vi "Untitled 1.vi"(7 "OPERACIONES":T2(ring), 8 "Error In":errorcluster, 10 "OPERADORES":T1 {"y 2" scale=0.0..4.0; "Meter" scale=-360.0..360.0 scale format="%#_3g"; "y" scale=-150.0..150.0; "x" scale=-150.0..150.0}, 11 "IMAGEN 1":path) -> (0 "Error Out":errorcluster, 1 "HISTOGRAMA":dbl[][](graph), 2 "IMAGEN MODIFICADA":picture, 3 "IMAGEN ORIGINAL":picture)   [LabVIEW 2016]
uses:
  <vilib>/picture/picture.llb/Draw True-Color Pixmap.vi
  <vilib>/imath/engines/lvmath2/RunTimeEngine/Managers/WorkSpace/UID Generator.vi
  <vilib>/imath/engines/lvmath2/RunTimeEngine/BuiltInFunctions/size/NIMS_[I32,I32]=size(GM).vi
  <instcachedir>/0/NIMS_[I32,I32]=size(GM)_B0A6EC1255BB4C8AB801FE6F734128D9.lvgen/NIMS_[I32,I32]=size(GM)_B0A6EC1255BB4C8AB801FE6F734128D9_005.vi
  <vilib>/imath/engines/lvmath2/RunTimeSupport/NIMS_Complex To Real.vi
  <instcachedir>/0/NIMS_Complex To Real_A9DD49CC305F495FA24B9F5762C73A31.lvgen/NIMS_Complex To Real_A9DD49CC305F495FA24B9F5762C73A31_001.vi
  <vilib>/imath/engines/lvmath2/RunTimeEngine/BuiltInFunctions/zeros/NIMS_M=zeros(I32,I32).vi
  <vilib>/imath/engines/lvmath2/RunTimeEngine/ErrorHandling/NIMS_Create Error From Enums.vi
  <vilib>/imath/engines/lvmath2/RunTimeEngine/RangeToken/NIMS_Range.vi
  <instcachedir>/0/NIMS_Range_A7C094595B484CA7AF10685B02D808ED.lvgen/NIMS_Range_A7C094595B484CA7AF10685B02D808ED_000.vi
  <vilib>/imath/engines/lvmath2/RunTimeSupport/NIMS_Error if Not Equal.vi
  <instcachedir>/0/NIMS_Error if Not Equal_43252A79AD05436189442EC0C5E5AB8A.lvgen/NIMS_Error if Not Equal_43252A79AD05436189442EC0C5E5AB8A_001.vi
  <vilib>/imath/engines/lvmath2/RunTimeEngine/IndexReplace/NIMS M(V,V)=M.vi
  <instcachedir>/0/NIMS M(V,V)=M_7C673E496ABD4677A4D7F51E7F4F45D1.lvgen/NIMS M(V,V)=M_7C673E496ABD4677A4D7F51E7F4F45D1_004.vi
  <vilib>/imath/engines/lvmath2/RunTimeEngine/BuiltInFunctions/size/NIMS_I32=size(GM,I32).vi
  <instcachedir>/0/NIMS_I32=size(GM,I32)_122058B1B3294FAEA5DC209B92B394E4.lvgen/NIMS_I32=size(GM,I32)_122058B1B3294FAEA5DC209B92B394E4_005.vi
  <vilib>/imathl/engines/lvmath/Functions/Error Handling/Create Error.vi
  <vilib>/imath/engines/lvmath2/RunTimeEngine/BuiltInFunctions/size/NIMS_I32Row=size(GM).vi
  <instcachedir>/0/NIMS_I32Row=size(GM)_10ACDCB9F1F84A7E9F42C91D87611FB5.lvgen/NIMS_I32Row=size(GM)_10ACDCB9F1F84A7E9F42C91D87611FB5_006.vi
  <vilib>/imath/engines/lvmath2/RunTimeEngine/BuiltInFunctions/zeros/NIMS_M=zeros(I32V).vi
  <vilib>/imath/engines/lvmath2/RunTimeEngine/RangeToken/NIMS_Range_R2 - Integer.vi
  <instcachedir>/0/NIMS_Range_R2 - Integer_89B873E74E6E489885E44F751DD9C6BF.lvgen/NIMS_Range_R2 - Integer_89B873E74E6E489885E44F751DD9C6BF_000.vi
  <vilib>/imath/engines/lvmath2/RunTimeEngine/CommandStatement/MC_CommandStatement_break.vi
  <vilib>/imath/engines/lvmath2/RunTimeEngine/BuiltInFunctions/round/NIMS_round(DBL-S).vi
  <instcachedir>/0/NIMS_Error if Not Equal_43252A79AD05436189442EC0C5E5AB8A.lvgen/NIMS_Error if Not Equal_43252A79AD05436189442EC0C5E5AB8A_000.vi
  <vilib>/imath/engines/lvmath2/RunTimeEngine/IndexRead/NIMS M(S,S).vi
  <instcachedir>/0/NIMS M(S,S)_AC51E74150A542F7991B9634C66F3096.lvgen/NIMS M(S,S)_AC51E74150A542F7991B9634C66F3096_002.vi
  <vilib>/imath/engines/lvmath2/RunTimeEngine/IndexReplace/NIMS M(S,S)=S.vi
  <instcachedir>/0/NIMS M(S,S)=S_98E40400474E4398B113AE20298B4F82.lvgen/NIMS M(S,S)=S_98E40400474E4398B113AE20298B4F82_003.vi
  <vilib>/imath/engines/lvmath2/RunTimeEngine/RunTimeType/NIMS_RunTimeType_From StrictType (excl LVString).vi
  <instcachedir>/0/NIMS_RunTimeType_From StrictType (excl LVString)_BBF44FB49F834B71AF7A14CCEDF8BECD.lvgen/NIMS_RunTimeType_From StrictType (excl LVString)_BBF44FB49F834B71AF7A14CCEDF8BECD_000.vi
  <vilib>/imath/engines/lvmath2/RunTimeEngine/LocalVariableDefStatement/MC_LocalVariableDefStatement_Display.vi
  <vilib>/imath/engines/lvmath2/RunTimeEngine/Managers/SymbolTable/Clear UID.vi
  <vilib>/imath/engines/lvmath2/RunTimeEngine/NodeEndStatement/NIMS_NodeEndStatement_Output.vi
  <instcachedir>/0/NIMS_NodeEndStatement_Output_53EC0D466D134D7ABD903AC30B43404B.lvgen/NIMS_NodeEndStatement_Output_53EC0D466D134D7ABD903AC30B43404B_001.vi
  <instcachedir>/0/NIMS_NodeEndStatement_Output_53EC0D466D134D7ABD903AC30B43404B.lvgen/NIMS_NodeEndStatement_Output_53EC0D466D134D7ABD903AC30B43404B_010.vi
  <vilib>/imath/engines/lvmath2/RunTimeEngine/ErrorHandling/NIMS_Finalize Error.vi
  <vilib>/Analysis/Matrix/Numeric/Conversions/Array To Matrix - RA2.vi
  <vilib>/Analysis/Matrix/Numeric/Conversions/Matrix To Array - RM.vi
  <vilib>/imath/engines/lvmath2/RunTimeEngine/BuiltInFunctions/rotate90/NIMS_rotate90.vi
  <instcachedir>/0/NIMS_rotate90_7DC1660D109944E092D2EB6E3185A1B6.lvgen/NIMS_rotate90_7DC1660D109944E092D2EB6E3185A1B6_004.vi
  <vilib>/imath/engines/lvmath2/RunTimeEngine/IndexRead/NIMS M(R2,S).vi
  <instcachedir>/0/NIMS M(R2,S)_56813DCFDD5A484292D2195AF15D2BF5.lvgen/NIMS M(R2,S)_56813DCFDD5A484292D2195AF15D2BF5_000.vi
  <vilib>/imath/engines/lvmath2/RunTimeEngine/IndexReplace/NIMS M(R2,S)=V.vi
  <instcachedir>/0/NIMS M(R2,S)=V_4CAA475A15784754AE70E3CCB958AE2E.lvgen/NIMS M(R2,S)=V_4CAA475A15784754AE70E3CCB958AE2E_000.vi
  <instcachedir>/0/NIMS_NodeEndStatement_Output_53EC0D466D134D7ABD903AC30B43404B.lvgen/NIMS_NodeEndStatement_Output_53EC0D466D134D7ABD903AC30B43404B_002.vi
  <instcachedir>/0/NIMS M(S,S)_AC51E74150A542F7991B9634C66F3096.lvgen/NIMS M(S,S)_AC51E74150A542F7991B9634C66F3096_003.vi
  <instcachedir>/0/NIMS M(S,S)_AC51E74150A542F7991B9634C66F3096.lvgen/NIMS M(S,S)_AC51E74150A542F7991B9634C66F3096_000.vi
  <instcachedir>/0/NIMS M(S,S)=S_98E40400474E4398B113AE20298B4F82.lvgen/NIMS M(S,S)=S_98E40400474E4398B113AE20298B4F82_000.vi
  <vilib>/Analysis/Matrix/NI_Matrix.lvlib
  <vilib>/imath/engines/lvmath2/RunTimeEngine/Managers/SymbolTable/NIMS_WorkSpace.lvlib
panel:
  out "size(s)":i32[](array[numeric])
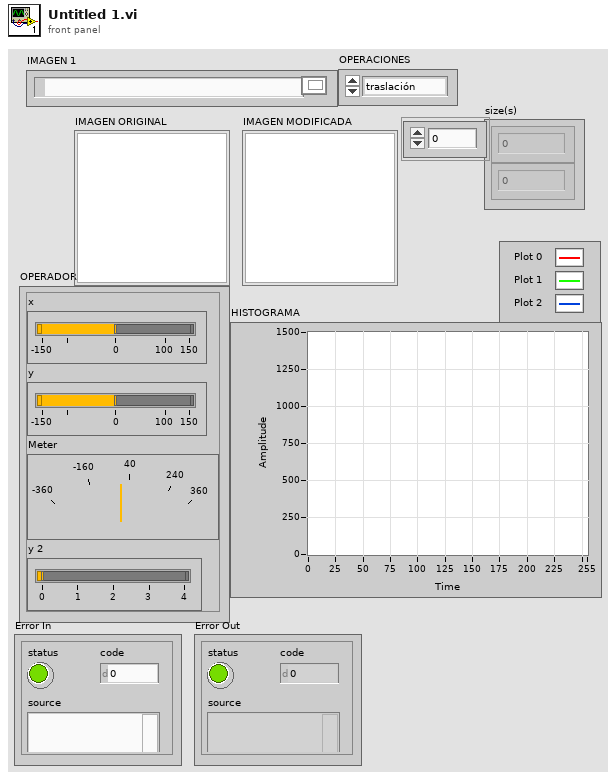
[diagram p1: front panel]
types:
  T1 = cluster{"x":dbl, "y":dbl, "Meter":dbl, "y 2":i64}
  T2 = enum16{"traslación", "Rotación", "Zoom", "GIROH", "GIROV", "Extracción", "Sustitución", "UNION"}
  T3 = typedef "imagedata.ctl" = cluster{"image type":i32, "image depth":i32, "image":u8[], "mask":u8[], "colors":u32[], "Rectangle":cluster{"left":i16, "top":i16, "right":i16, "bottom":i16}}
  T4 = typedef "NI_Matrix.lvlib/RealMatrix.ctl" = dbl[][]
  T5 = cluster{"left":i16, "top":i16, "right":i16, "bottom":i16}
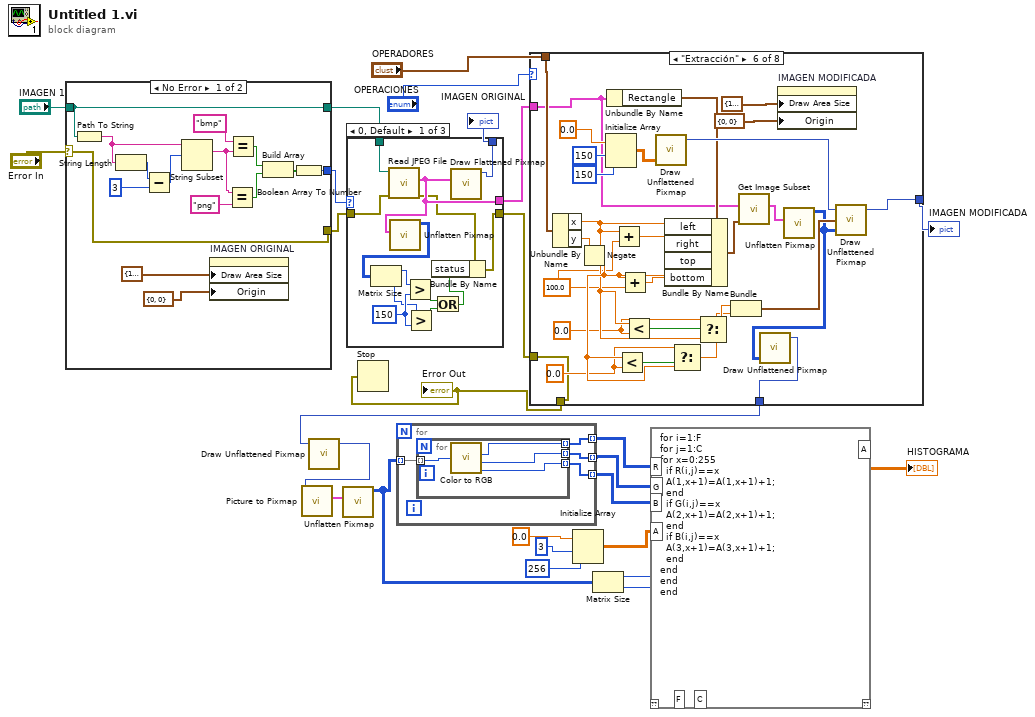
[diagram p0: block diagram]
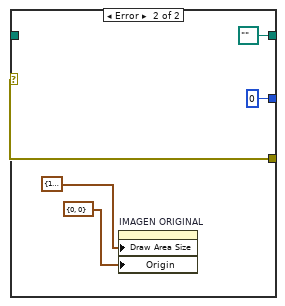
[diagram p2: hidden frame]
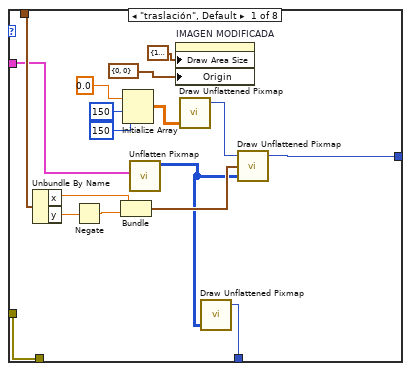
[diagram p3: hidden frame]
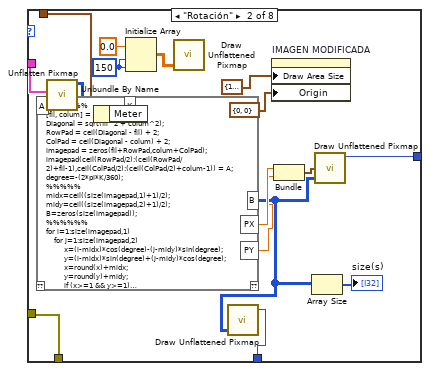
[diagram p4: hidden frame]
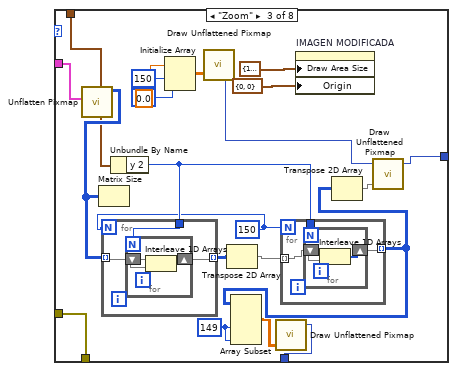
[diagram p5: hidden frame]
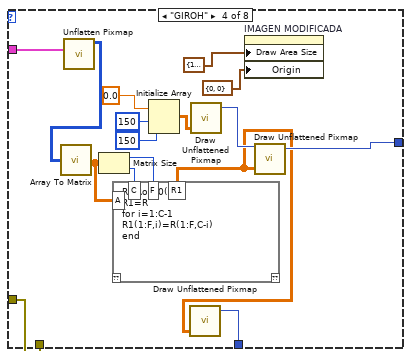
[diagram p6: hidden frame]
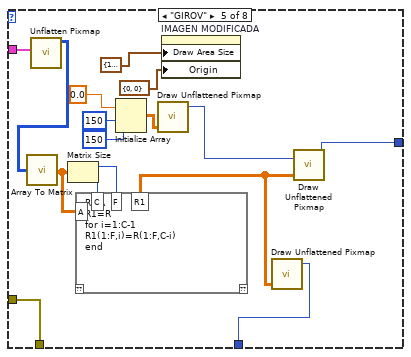
[diagram p7: hidden frame]
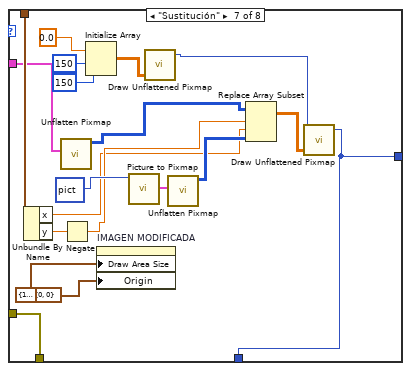
[diagram p8: hidden frame]
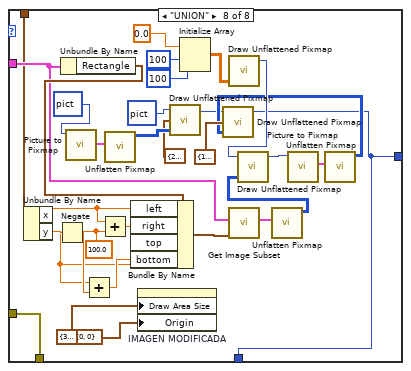
[diagram p9: hidden frame]
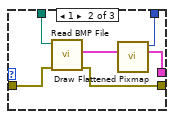
[diagram p10: hidden frame]
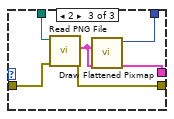
[diagram p11: hidden frame]
diagram:
  n1 = case shown="No Error" "Error In" {
    selector: "Error In" -> [w30 w46]
    tunnel: [w36 u32 0] -> w26
    tunnel: [w29 path "" ("File Path Control")] -> w25
    tunnel: [w30 w46] -> w24
    tunnel: "IMAGEN 1" -> [w29 _]
    frame No Error {
      n2 = Path To String(path=w29) -> (string=w31:string)
      n3 = String Length(string=w31) -> (length=w41:i32)
      n4 = Subtract(x=w41, y=3) -> (x-y=w39:i32)
      n5 = String Subset(string=w31, offset (0)=w39) -> (substring=w32:string)  [unwired: 1 in]
      n6 = property on="IMAGEN ORIGINAL" class="Pict"("Draw Area Size"=cluster{"Width":u32, "Height":u32} {"Width"=150, "Height"=150} ("Caption.Size"), "Origin"=cluster{"Horizontal":i16, "Vertical":i16} {"Horizontal"=0, "Vertical"=0}) -> ()  [unwired: 2 in, 2 out]
      n7 = Equal?(x=w32, y="png" ("x")) -> (x = y?=w34:bool)
      n8 = Equal?(x="bmp", y=w32) -> (x = y?=w33:bool)
      n9 = Build Array(w33, w34) -> (w35:bool[])
      n10 = Boolean Array To Number(Boolean array=w35) -> (number=w36:u32)
    }
    frame Error {
      n11 = property on="IMAGEN ORIGINAL" class="Pict"("Draw Area Size"=cluster{"Width":u32, "Height":u32} {"Width"=150, "Height"=150} ("Caption.Size"), "Origin"=cluster{"Horizontal":i16, "Vertical":i16} {"Horizontal"=0, "Vertical"=0}) -> ()  [unwired: 2 in, 2 out]
    }
  }
  n12 = case shown="0, Default" w26 {
    tunnel: w25 -> [w59 w64 w69]
    tunnel: [w56 w63 w68] -> w21
    tunnel: w24 -> [w58 w62 w67]
    tunnel: [w47 w61 w66] -> w16
    tunnel: [w57 w60 w65] -> w20
    frame 0, Default {
      w52 = 150 ("y")
      n13 = call <vilib>:"Read JPEG File.vi"("error in (no error)"=w58, "path to JPEG file"=w59) -> ("error out"=w48:errorcluster, "image data"=w56:T3)  [unwired: 7 in, 1 out]
      n14 = call <vilib>:"Unflatten Pixmap.vi"("image data"=w56) -> ("24-bit pixmap"=w55:u32[][])  [unwired: 4 in, 6 out]
      n15 = Matrix Size(0:w55) -> (1:w51:i32, 2:w50:i32)
      n16 = Greater?(x=w51, y=w52) -> (0:w53:bool)
      n17 = Greater?(x=w50, y=w52) -> (0:w54:bool)
      n18 = Or(x=w53, y=w54) -> (x .or. y?=w49:bool)
      n19 = Bundle By Name(cluster=w48, "status"=w49) -> (w47:errorcluster)
      n20 = call <vilib>:"Draw Flattened Pixmap.vi"("image data"=w56) -> ("new picture"=w57:picture)  [unwired: 8 in]
    }
    frame 1 {
      n21 = call <vilib>:"Read BMP File.vi"("error in (no error)"=w62, "path to BMP file"=w64) -> ("error out"=w61:errorcluster, "image data"=w63:T3)  [unwired: 7 in, 1 out]
      n22 = call <vilib>:"Draw Flattened Pixmap.vi"("image data"=w63) -> ("new picture"=w60:picture)  [unwired: 8 in]
    }
    frame 2 {
      n23 = call <vilib>:"Read PNG File.vi"("error in (no error)"=w67, "path to PNG file"=w69) -> ("error out"=w66:errorcluster, "image data"=w68:T3)  [unwired: 7 in, 1 out]
      n24 = call <vilib>:"Draw Flattened Pixmap.vi"("image data"=w68) -> ("new picture"=w65:picture)  [unwired: 8 in]
    }
  }
  "IMAGEN ORIGINAL" <- w20
  n25 = case shown="\"Extracción\"" "OPERACIONES" {
    tunnel: [w83 w103 w633 w663 w828 w966 w995 w1012] -> w19
    tunnel: w21 -> [w78 w101 w634 w662 w822 w967 w1002 w1040]
    tunnel: "OPERADORES" -> [w80 w102 w635 _ _ w968 w1011 w1036]
    tunnel: w16 -> [w77 w98 w647 w673 w815 w969 w1001 w1013]
    tunnel: [w77 w98 w647 w673 w815 w969 w1001 w1013] -> w15
    tunnel: [w70 w92 w632 w660 w813 w964 w995 w1012] -> w14
    frame "traslación", Default {
      n26 = Unbundle By Name(w80) -> ("x"=w79:dbl, "y"=w74:dbl)
      n27 = Negate(x=w74) -> (-x=w73:dbl)
      n28 = Bundle("x"=w79, w73) -> (w72:cluster{"x":dbl, dbl})  [unwired: 1 in]
      n29 = Initialize Array(0.0 ("element"), 150 ("dimension size"), 150 ("dimension size")) -> (w82:dbl[][])
      n30 = call <vilib>:"Unflatten Pixmap.vi"("image data"=w78) -> ("24-bit pixmap"=w71:u32[][])  [unwired: 4 in, 6 out]
      n31 = property on="IMAGEN MODIFICADA" class="Pict"("Draw Area Size"=cluster{"Width":u32, "Height":u32} {"Width"=150, "Height"=150} ("Caption.Size"), "Origin"=cluster{"Horizontal":i16, "Vertical":i16} {"Horizontal"=0, "Vertical"=0}) -> ()  [unwired: 2 in, 2 out]
      n32 = call-poly <vilib>:"Draw Unflattened Pixmap.vi"("data (RGB format)"=w82) -> ("new picture"=w81:picture)  [unwired: 8 in]
      n33 = call-poly <vilib>:"Draw Unflattened Pixmap.vi"("data (RGB format)"=w71) -> ("new picture"=w70:picture)  [unwired: 8 in]
      n34 = call-poly <vilib>:"Draw Unflattened Pixmap.vi"("picture"=w81, "top left point(0, 0)"=w72, "data (RGB format)"=w71) -> ("new picture"=w83:picture)  [unwired: 6 in]
    }
    frame "Rotación" {
      w97 = 150 ("dimension size")
      n35 = call <vilib>:"Unflatten Pixmap.vi"("image data"=w101) -> ("24-bit pixmap"=w93:u32[][])  [unwired: 4 in, 6 out]
      n36 = Unbundle By Name(w102) -> ("Meter"=w94:dbl)
      n37 = mathscript code="%%%%%%\n[fil, colum] = size(A); \nDiagonal = sqrt(fil^2 + colum^2); \nRowPad = ceil(Diagonal - fil) + 2;\nColPad = ceil(Diagonal - colum) + 2;\nimagepad = zeros(fil+RowPad,colum+ColPad);\nimagepad(ceil(RowPad/2):(ceil(RowPad/2)+fil-1),ceil(ColPad/2):(ceil(ColPad/2)+colum-1)) = A;\ndegree=-(2*pi*K/360);\n%%%%%\nmidx=ceil((size(imagepad,1)+1)/2);\nmidy=ceil((size(imagepad,2)+1)/2);\nB=zeros(size(imagepad));\n%%%%%%\nfor i=1:size(imagepad,1)\n    for j=1:size(imagepad,2)\n         x=(i-midx)*cos(degree)-(j-midy)*sin(degree);\n         y=(i-midx)*sin(degree)+(j-midy)*cos(degree);\n         x=round(x)+midx;\n         y=round(y)+midy;\n         if (x>=1 && y>=1)\n             B(x,y)=imagepad(i,j);        \n         end\n    end\nend\n[m,n]=size(B)\nPY=-(midy/2)-2\nPX=-(midx/8)-2"("K"=w94, "A"=w93) -> ("B"=w88:u32[][], "PX"=w90:dbl, "PY"=w89:dbl)  [unwired: 1 in, 1 out]
      n38 = Initialize Array(0.0 ("element"), w97, w97) -> (w95:dbl[][])
      n39 = call-poly <vilib>:"Draw Unflattened Pixmap.vi"("data (RGB format)"=w95) -> ()  [unwired: 8 in, 1 out]
      n40 = call-poly <vilib>:"Draw Unflattened Pixmap.vi"("data (RGB format)"=w88) -> ("new picture"=w92:picture)  [unwired: 8 in]
      n41 = property on="IMAGEN MODIFICADA" class="Pict"("Draw Area Size"=cluster{"Width":u32, "Height":u32} {"Width"=150, "Height"=150} ("Caption.Size"), "Origin"=cluster{"Horizontal":i16, "Vertical":i16} {"Horizontal"=0, "Vertical"=0}) -> ()  [unwired: 2 in, 2 out]
      n42 = Bundle("PX"=w90, "PY"=w89) -> (w91:cluster{"PX":dbl, "PY":dbl})  [unwired: 1 in]
      n43 = Array Size(array=w88) -> (size(s)=→"size(s)":i32[])
      n44 = call-poly <vilib>:"Draw Unflattened Pixmap.vi"("top left point(0, 0)"=w91, "data (RGB format)"=w88) -> ("new picture"=w103:picture)  [unwired: 7 in]
    }
    frame "Zoom" {
      w629 = 149 ("row N")
      w637 = 150
      n45 = call <vilib>:"Unflatten Pixmap.vi"("image data"=w634) -> ("24-bit pixmap"=w636:u32[][])  [unwired: 4 in, 6 out]
      n46 = Matrix Size(0:w636) -> ()  [unwired: 2 out]
      n47 = Unbundle By Name(w635) -> ("y 2"=w639:i64)
      n48 = for {
        N: w637 -> [_]
        tunnel: w636 -> [w657] mode=indexing
        tunnel: w639 -> [w656]
        tunnel: [w655] -> w641 mode=indexing
        n49 = for {
          N: w656 -> [_]
          shift-right: [w658] -> w655
          shift-left: w657 -> [w659]
          n50 = Interleave 1D Arrays(w659, w659) -> (w658:u32[])
        }
      }
      n51 = Initialize Array(0.0 ("element"), 150 ("dimension size"), 150 ("dimension size")) -> (w643:dbl[][])
      n52 = call-poly <vilib>:"Draw Unflattened Pixmap.vi"("data (RGB format)"=w643) -> ("new picture"=w642:picture)  [unwired: 8 in]
      n53 = Transpose 2D Array(2D array=w641) -> (transposed array=w640:u32[][])
      n54 = for {
        N: w637 -> [_]
        tunnel: w639 -> [w652]
        tunnel: [w651] -> w631 mode=indexing
        tunnel: w640 -> [w650] mode=indexing
        n55 = for {
          N: w652 -> [_]
          shift-right: [w653] -> w651
          shift-left: w650 -> [w654]
          n56 = Interleave 1D Arrays(w654, w654) -> (w653:u32[])
        }
      }
      n57 = Array Subset(array=w631, length (row)=w629, length (col)=w629) -> (w630:dbl[][])  [unwired: 2 in]
      n58 = call-poly <vilib>:"Draw Unflattened Pixmap.vi"("data (RGB format)"=w630) -> ("new picture"=w632:picture)  [unwired: 8 in]
      n59 = property on="IMAGEN MODIFICADA" class="Pict"("Draw Area Size"=cluster{"Width":u32, "Height":u32} {"Width"=150, "Height"=150} ("Caption.Size"), "Origin"=cluster{"Horizontal":i16, "Vertical":i16} {"Horizontal"=0, "Vertical"=0}) -> ()  [unwired: 2 in, 2 out]
      n60 = Transpose 2D Array(2D array=w631) -> (transposed array=w638:u32[][])
      n61 = call-poly <vilib>:"Draw Unflattened Pixmap.vi"("picture"=w642, "data (RGB format)"=w638) -> ("new picture"=w633:picture)  [unwired: 7 in]
    }
    frame "GIROH" {
      n62 = call <vilib>:"Unflatten Pixmap.vi"("image data"=w662) -> ("24-bit pixmap"=w667:u32[][])  [unwired: 4 in, 6 out]
      n63 = call-poly <vilib>:"Array To Matrix.vi"("Real 2D Array"=w667) -> ("Real Matrix"=w664:T4)
      n64 = Matrix Size(0:w664) -> (1:w665:i32, 2:w672:i32)
      n65 = mathscript code="R=Rot90(A,2)\nR1=R\nfor i=1:C-1\nR1(1:F,i)=R(1:F,C-i)\nend"("A"=w664, "C"=w672, "F"=w665) -> ("R1"=w661:dbl[][])  [unwired: 1 in, 1 out]
      n66 = Initialize Array(0.0 ("element"), 150 ("dimension size"), 150 ("dimension size")) -> (w668:dbl[][])
      n67 = call-poly <vilib>:"Draw Unflattened Pixmap.vi"("data (RGB format)"=w661) -> ("new picture"=w660:picture)  [unwired: 8 in]
      n68 = call-poly <vilib>:"Draw Unflattened Pixmap.vi"("data (RGB format)"=w668) -> ("new picture"=w666:picture)  [unwired: 8 in]
      n69 = property on="IMAGEN MODIFICADA" class="Pict"("Draw Area Size"=cluster{"Width":u32, "Height":u32} {"Width"=150, "Height"=150} ("Caption.Size"), "Origin"=cluster{"Horizontal":i16, "Vertical":i16} {"Horizontal"=0, "Vertical"=0}) -> ()  [unwired: 2 in, 2 out]
      n70 = call-poly <vilib>:"Draw Unflattened Pixmap.vi"("picture"=w666, "data (RGB format)"=w661) -> ("new picture"=w663:picture)  [unwired: 7 in]
    }
    frame "GIROV" {
      n71 = call <vilib>:"Unflatten Pixmap.vi"("image data"=w822) -> ("24-bit pixmap"=w821:u32[][])  [unwired: 4 in, 6 out]
      n72 = call-poly <vilib>:"Array To Matrix.vi"("Real 2D Array"=w821) -> ("Real Matrix"=w818:T4)
      n73 = Matrix Size(0:w818) -> (1:w819:i32, 2:w827:i32)
      n74 = mathscript code="R=A\nR1=R\nfor i=1:C-1\nR1(1:F,i)=R(1:F,C-i)\nend"("A"=w818, "C"=w827, "F"=w819) -> ("R1"=w814:dbl[][])  [unwired: 1 in, 1 out]
      n75 = Initialize Array(0.0 ("element"), 150 ("dimension size"), 150 ("dimension size")) -> (w823:dbl[][])
      n76 = call-poly <vilib>:"Draw Unflattened Pixmap.vi"("data (RGB format)"=w823) -> ("new picture"=w820:picture)  [unwired: 8 in]
      n77 = property on="IMAGEN MODIFICADA" class="Pict"("Draw Area Size"=cluster{"Width":u32, "Height":u32} {"Width"=150, "Height"=150} ("Caption.Size"), "Origin"=cluster{"Horizontal":i16, "Vertical":i16} {"Horizontal"=0, "Vertical"=0}) -> ()  [unwired: 2 in, 2 out]
      n78 = call-poly <vilib>:"Draw Unflattened Pixmap.vi"("data (RGB format)"=w814) -> ("new picture"=w813:picture)  [unwired: 8 in]
      n79 = call-poly <vilib>:"Draw Unflattened Pixmap.vi"("picture"=w820, "data (RGB format)"=w814) -> ("new picture"=w828:picture)  [unwired: 7 in]
    }
    frame "Extracción" {
      w987 = 0.0 ("y")
      w986 = 0.0 ("y")
      w982 = 100.0 ("y")
      n80 = Unbundle By Name(w968) -> ("x"=w991:dbl, "y"=w984:dbl)
      n81 = Negate(x=w984) -> (-x=w992:dbl)
      n82 = Initialize Array(0.0 ("element"), 150 ("dimension size"), 150 ("dimension size")) -> (w978:dbl[][])
      n83 = Unbundle By Name(w967) -> ("Rectangle"=w970:T5)
      n84 = Add(x=w991, y=w982) -> (x+y=w973:dbl)
      n85 = Less?(x=w992, y=w986) -> (x < y?=w983:bool)
      n86 = Add(x=w992, y=w982) -> (x+y=w972:dbl)
      n87 = Less?(x=w991, y=w987) -> (x < y?=w988:bool)
      n88 = call-poly <vilib>:"Draw Unflattened Pixmap.vi"("data (RGB format)"=w978) -> ("new picture"=w979:picture)  [unwired: 8 in]
      n89 = Bundle By Name(cluster=w970, "left"=w991, "right"=w973, "top"=w992, "bottom"=w972) -> (w971:T5)
      n90 = Select(t=w986, s=w983, f=w992) -> (s? t:f=w985:dbl)
      n91 = Select(t=w987, s=w988, f=w991) -> (s? t:f=w989:dbl)
      n92 = Bundle("x"=w989, "y"=w985) -> (w990:cluster{"x":dbl, "y":dbl})  [unwired: 1 in]
      n93 = call <vilib>:"Get Image Subset.vi"("subset rect"=w971, "image data"=w967) -> ("image subset"=w974:T3)  [unwired: 4 in, 1 out]
      n94 = property on="IMAGEN MODIFICADA" class="Pict"("Draw Area Size"=cluster{"Width":u32, "Height":u32} {"Width"=150, "Height"=150} ("Caption.Size"), "Origin"=cluster{"Horizontal":i16, "Vertical":i16} {"Horizontal"=0, "Vertical"=0}) -> ()  [unwired: 2 in, 2 out]
      n95 = call <vilib>:"Unflatten Pixmap.vi"("image data"=w974) -> ("24-bit pixmap"=w965:u32[][])  [unwired: 4 in, 6 out]
      n96 = call-poly <vilib>:"Draw Unflattened Pixmap.vi"("data (RGB format)"=w965) -> ("new picture"=w964:picture)  [unwired: 8 in]
      n97 = call-poly <vilib>:"Draw Unflattened Pixmap.vi"("picture"=w979, "top left point(0, 0)"=w990, "data (RGB format)"=w965) -> ("new picture"=w966:picture)  [unwired: 6 in]
    }
    frame "Sustitución" {
      n98 = Unbundle By Name(w1011) -> ("x"=w993:dbl, "y"=w1007:dbl)
      n99 = call <vilib>:"Unflatten Pixmap.vi"("image data"=w1002) -> ("24-bit pixmap"=w999:u32[][])  [unwired: 4 in, 6 out]
      n100 = Negate(x=w1007) -> (-x=w994:dbl)
      n101 = Initialize Array(0.0 ("element"), 150 ("dimension size"), 150 ("dimension size")) -> (w1003:dbl[][])
      n102 = property on="IMAGEN MODIFICADA" class="Pict"("Draw Area Size"=cluster{"Width":u32, "Height":u32} {"Width"=150, "Height"=150} ("Caption.Size"), "Origin"=cluster{"Horizontal":i16, "Vertical":i16} {"Horizontal"=0, "Vertical"=0}) -> ()  [unwired: 2 in, 2 out]
      n103 = call <vilib>:"Picture to Pixmap.vi"("picture"=picture bytes[30030] ("IMAGEN ORIGINAL 2")) -> ("image data"=w1006:T3)  [unwired: 9 in, 1 out]
      n104 = call-poly <vilib>:"Draw Unflattened Pixmap.vi"("data (RGB format)"=w1003) -> ("new picture"=w996:picture)  [unwired: 8 in]
      n105 = call <vilib>:"Unflatten Pixmap.vi"("image data"=w1006) -> ("24-bit pixmap"=w998:u32[][])  [unwired: 4 in, 6 out]
      n106 = Replace Array Subset(array=w999, new element=w998, index (row)=w994, index (col)=w993) -> (w997:T4)
      n107 = call-poly <vilib>:"Draw Unflattened Pixmap.vi"("picture"=w996, "data (RGB format)"=w997) -> ("new picture"=w995:picture)  [unwired: 7 in]
    }
    frame "UNION" {
      w1031 = 100.0 ("y")
      n108 = Unbundle By Name(w1036) -> ("x"=w1022:dbl, "y"=w1030:dbl)
      n109 = Negate(x=w1030) -> (-x=w1023:dbl)
      n110 = Unbundle By Name(w1040) -> ("Rectangle"=w1042:T5)
      n111 = call <vilib>:"Picture to Pixmap.vi"("picture"=picture bytes[30030] ("new picture 3")) -> ("image data"=w1029:T3)  [unwired: 9 in, 1 out]
      n112 = Add(x=w1023, y=w1031) -> (x+y=w1039:dbl)
      n113 = Add(x=w1022, y=w1031) -> (x+y=w1038:dbl)
      n114 = call <vilib>:"Unflatten Pixmap.vi"("image data"=w1029) -> ("24-bit pixmap"=w1028:u32[][])  [unwired: 4 in, 6 out]
      n115 = Bundle By Name(cluster=w1042, "left"=w1022, "right"=w1038, "top"=w1023, "bottom"=w1039) -> (w1041:T5)
      n116 = property on="IMAGEN MODIFICADA" class="Pict"("Draw Area Size"=cluster{"Width":u32, "Height":u32} {"Width"=300, "Height"=100} ("Caption.Size"), "Origin"=cluster{"Horizontal":i16, "Vertical":i16} {"Horizontal"=0, "Vertical"=0}) -> ()  [unwired: 2 in, 2 out]
      n117 = call-poly <vilib>:"Draw Unflattened Pixmap.vi"("picture"=picture bytes[30030] ("new picture 3"), "top left point(0, 0)"=cluster{"x":i16, "y":i16} {"x"=200, "y"=0}, "data (RGB format)"=w1028) -> ("new picture"=w1014:picture)  [unwired: 6 in]
      n118 = Initialize Array(0.0 ("element"), 100 ("dimension size"), 100 ("dimension size")) -> (w1032:dbl[][])
      n119 = call-poly <vilib>:"Draw Unflattened Pixmap.vi"("data (RGB format)"=w1032) -> ("new picture"=w1017:picture)  [unwired: 8 in]
      n120 = call <vilib>:"Get Image Subset.vi"("subset rect"=w1041, "image data"=w1040) -> ("image subset"=w1037:T3)  [unwired: 4 in, 1 out]
      n121 = call <vilib>:"Unflatten Pixmap.vi"("image data"=w1037) -> ("24-bit pixmap"=w1018:u32[][])  [unwired: 4 in, 6 out]
      n122 = call-poly <vilib>:"Draw Unflattened Pixmap.vi"("picture"=w1017, "data (RGB format)"=w1018) -> ("new picture"=w1016:picture)  [unwired: 7 in]
      n123 = call <vilib>:"Picture to Pixmap.vi"("picture"=w1016) -> ("image data"=w1026:T3)  [unwired: 9 in, 1 out]
      n124 = call <vilib>:"Unflatten Pixmap.vi"("image data"=w1026) -> ("24-bit pixmap"=w1015:u32[][])  [unwired: 4 in, 6 out]
      n125 = call-poly <vilib>:"Draw Unflattened Pixmap.vi"("picture"=w1014, "top left point(0, 0)"=cluster{"x":i16, "y":i16} {"x"=100, "y"=0}, "data (RGB format)"=w1015) -> ("new picture"=w1012:picture)  [unwired: 6 in]
    }
  }
  "Error Out" <- w15
  "IMAGEN MODIFICADA" <- w19
  n126 = call-poly <vilib>:"Draw Unflattened Pixmap.vi"("picture"=w14) -> ("new picture"=w12:picture)  [unwired: 8 in]
  n127 = call <vilib>:"Picture to Pixmap.vi"("picture"=w12) -> ("image data"=w11:T3)  [unwired: 9 in, 1 out]
  n128 = call <vilib>:"Unflatten Pixmap.vi"("image data"=w11) -> ("24-bit pixmap"=w3:u32[][])  [unwired: 4 in, 6 out]
  n129 = Stop(stop? (T)=w15) -> ()
  n130 = for {
    tunnel: w3 -> [w1046] mode=indexing
    tunnel: [w1045] -> w9 mode=indexing
    tunnel: [w1044] -> w4 mode=indexing
    tunnel: [w1043] -> w8 mode=indexing
    n131 = for {
      tunnel: w1046 -> [w1050] mode=indexing
      tunnel: [w1049] -> w1045 mode=indexing
      tunnel: [w1048] -> w1044 mode=indexing
      tunnel: [w1047] -> w1043 mode=indexing
      n132 = call <vilib>:"Color to RGB.vi"("Color"=w1050) -> ("R"=w1049:u8, "G"=w1048:u8, "B"=w1047:u8)  [unwired: 1 out]
    }
  }
  n133 = Initialize Array(0.0 ("element"), 3 ("dimension size"), 256 ("dimension size")) -> (w5:dbl[][])
  n134 = Matrix Size(0:w3) -> (1:w2:i32, 2:w1:i32)
  n135 = mathscript code="for i=1:F\nfor j=1:C\nfor x=0:255\n  if R(i,j)==x\n  A(1,x+1)=A(1,x+1)+1;\n  end\n  if G(i,j)==x\n  A(2,x+1)=A(2,x+1)+1;\n  end\n  if B(i,j)==x\n  A(3,x+1)=A(3,x+1)+1;\n  end\nend\nend\nend"("R"=w9, "A"=w5, "G"=w4, "B"=w8, "F"=w2, "C"=w1) -> ("A"=→"HISTOGRAMA":dbl[][])  [unwired: 1 in, 1 out]
